vi "Write Pin simulated.vi"(8 "error in (no error)":errorcluster, 9 "1/0":bool, 10 "Pin":dbl, 11 "Simulated Device in":refnum<class "Simulated Device.lvclass">) -> (0 "error out":errorcluster, 2 "Read":string, 3 "Simulated Device out":refnum<class "Simulated Device.lvclass">)   [LabVIEW 2020, in "Simulated Device.lvclass"]
uses:
  Simulated Device.lvclass
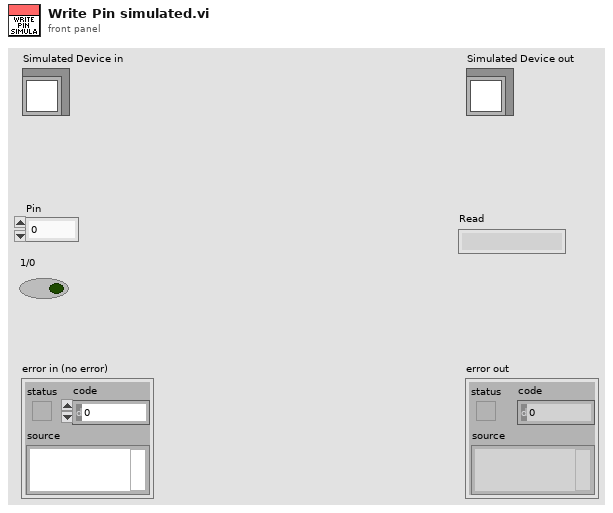
[diagram p1: front panel]
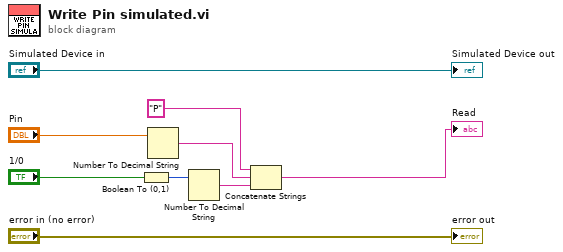
[diagram p0: block diagram]
diagram:
  n1 = Boolean To (0,1)(Boolean="1/0") -> (0, 1=w7:i16)
  n2 = Number To Decimal String(number="Pin") -> (decimal integer string=w5:string)  [unwired: 1 in]
  n3 = Number To Decimal String(number=w7) -> (decimal integer string=w6:string)  [unwired: 1 in]
  n4 = Concatenate Strings("P" ("string"), w5, w6) -> (→"Read":string)
  "error out" <- "error in (no error)"
  "Simulated Device out" <- "Simulated Device in"
